vi "canDataSort.vi"() -> ()   [LabVIEW 2023] (continued)
FF\tFF\tFF\tFF\t8C\r\n      1392  1FFFFFFF   00000004    8        00\t00\tFF\tFF\tFF\tFF\tFF\tFF\r\n      1383  0CF102A7   00000004    8        30\t75\tE0\t2E\t80\tFF\tFF\tFD\r\n      1383  0CF101A7   00000004    8        68\t00\t97\tCC\t00\t16\t39\t5F\r\n      1382  1FFFFFFF   00000004    8        00\t00\tFF\tFF\tFF\tFF\tFF\tFF\r\n      1372  1FFFFFFF   00000004    8        00\t00\tFF\tFF\tFF\tFF\tFF\tFF\r\n      1363  0CF102A7   00000004    8        30\t75\tE0\t2E\t80\tFF\tFF\tFD\r\n      1363  0CF101A7   00000004    8        68\t00\t97\tCC\t00\t16\t39\t5E\r\n      1362  1FFFFFFF   00000004    8        00\t00\tFF\tFF\tFF\tFF\tFF\tFF\r\n      1403  0CF102A7   00000004    8        30\t75\tE0\t2E\t80\tFF\tFF\tFD\r\n      1403  0CF101A7   00000004    8        68\t00\t97\tCC\t00\t16\t39\t60\r\n      1402  1FFFFFFF   00000004    8        00\t00\tFF\tFF\tFF\tFF\tFF\tFF\r\n      1393  18F106A7   00000004    8        00\tF7\tFF\tFF\tFF\tFF\tFF\t8C\r\n      1392  1FFFFFFF   00000004    8        00\t00\tFF\tFF\tFF\tFF\tFF\tFF\r\n      1383  0CF102A7   00000004    8        30\t75\tE0\t2E\t80\tFF\tFF\tFD\r\n      1383  0CF101A7   00000004    8        68\t00\t97\tCC\t00\t16\t39\t5F\r\n      1382  1FFFFFFF   00000004    8        00\t00\tFF\tFF\tFF\tFF\tFF\tFF\r\n      1372  1FFFFFFF   00000004    8        00\t00\tFF\tFF\tFF\tFF\tFF\tFF\r\n      1363  0CF102A7   00000004    8        30\t75\tE0\t2E\t80\tFF\tFF\tFD\r\n      1363  0CF101A7   00000004    8        68\t00\t97\tCC\t00\t16\t39\t5E\r\n      1412  1FFFFFFF   00000004    8        00\t00\tFF\tFF\tFF\tFF\tFF\tFF\r\n      1403  0CF102A7   00000004    8        30\t75\tE0\t2E\t80\tFF\tFF\tFD\r\n      1403  0CF101A7   00000004    8        68\t00\t97\tCC\t00\t16\t39\t60\r\n      1402  1FFFFFFF   00000004    8        00\t00\tFF\tFF\tFF\tFF\tFF\tFF\r\n      1393  18F106A7   00000004    8        00\tF7\tFF\tFF\tFF\tFF\tFF\t8C\r\n      1392  1FFFFFFF   00000004    8        00\t00\tFF\tFF\tFF\tFF\tFF\tFF\r\n      1383  0CF102A7   00000004    8        30\t75\tE0\t2E\t80\tFF\tFF\tFD\r\n      1383  0CF101A7   00000004    8        68\t00\t97\tCC\t00\t16\t39\t5F\r\n      1382  1FFFFFFF   00000004    8        00\t00\tFF\tFF\tFF\tFF\tFF\tFF\r\n      1372  1FFFFFFF   00000004    8        00\t00\tFF\tFF\tFF\tFF\tFF\tFF\r\n      1363  0CF102A7   00000004    8        30\t75\tE0\t2E\t80\tFF\tFF\tFD\r\n      1422  1FFFFFFF   00000004    8        00\t00\tFF\tFF\tFF\tFF\tFF\tFF\r\n      1412  1FFFFFFF   00000004    8        00\t00\tFF\tFF\tFF\tFF\tFF\tFF\r\n      1403  0CF102A7   00000004    8        30\t75\tE0\t2E\t80\tFF\tFF\tFD\r\n      1403  0CF101A7   00000004    8        68\t00\t97\tCC\t00\t16\t39\t60\r\n      1402  1FFFFFFF   00000004    8        00\t00\tFF\tFF\tFF\tFF\tFF\tFF\r\n      1393  18F106A7   00000004    8        00\tF7\tFF\tFF\tFF\tFF\tFF\t8C\r\n      1392  1FFFFFFF   00000004    8        00\t00\tFF\tFF\tFF\tFF\tFF\tFF\r\n      1383  0CF102A7   00000004    8        30\t75\tE0\t2E\t80\tFF\tFF\tFD\r\n      1383  0CF101A7   00000004    8        68\t00\t97\tCC\t00\t16\t39\t5F\r\n      1382  1FFFFFFF   00000004    8        00\t00\tFF\tFF\tFF\tFF\tFF\tFF\r\n      1372  1FFFFFFF   00000004    8        00\t00\tFF\tFF\tFF\tFF\tFF\tFF\r\n      1423  0CF101A7   00000004    8        68\t00\t97\tCC\t00\t16\t39\t61\r\n      1422  1FFFFFFF   00000004    8        00\t00\tFF\tFF\tFF\tFF\tFF\tFF\r\n      1412  1FFFFFFF   00000004    8        00\t00\tFF\tFF\tFF\tFF\tFF\tFF\r\n      1403  0CF102A7   00000004    8        30\t75\tE0\t2E\t80\tFF\tFF\tFD\r\n      1403  0CF101A7   00000004    8        68\t00\t97\tCC\t00\t16\t39\t60\r\n      1402  1FFFFFFF   00000004    8        00\t00\tFF\tFF\tFF\tFF\tFF\tFF\r\n      1393  18F106A7   00000004    8        00\tF7\tFF\tFF\tFF\tFF\tFF\t8C\r\n      1392  1FFFFFFF   00000004    8        00\t00\tFF\tFF\tFF\tFF\tFF\tFF\r\n      1383  0CF102A7   00000004    8        30\t75\tE0\t2E\t80\tFF\tFF\tFD\r\n      1383  0CF101A7   00000004    8        68\t00\t97\tCC\t00\t16\t39\t5F\r\n      1382  1FFFFFFF   00000004    8        00\t00\tFF\tFF\tFF\tFF\tFF\tFF\r\n      1423  0CF102A7   00000004    8        30\t75\tE0\t2E\t80\tFF\tFF\tFD\r\n      1423  0CF101A7   00000004    8        68\t00\t97\tCC\t00\t16\t39\t61\r\n      1422  1FFFFFFF   00000004    8        00\t00\tFF\tFF\tFF\tFF\tFF\tFF\r\n      1412  1FFFFFFF   00000004    8        00\t00\tFF\tFF\tFF\tFF\tFF\tFF\r\n      1403  0CF102A7   00000004    8        30\t75\tE0\t2E\t80\tFF\tFF\tFD\r\n      1403  0CF101A7   00000004    8        68\t00\t97\tCC\t00\t16\t39\t60\r\n      1402  1FFFFFFF   00000004    8        00\t00\tFF\tFF\tFF\tFF\tFF\tFF\r\n      1393  18F106A7   00000004    8        00\tF7\tFF\tFF\tFF\tFF\tFF\t8C\r\n      1392  1FFFFFFF   00000004    8        00\t00\tFF\tFF\tFF\tFF\tFF\tFF\r\n      1383  0CF102A7   00000004    8        30\t75\tE0\t2E\t80\tFF\tFF\tFD\r\n      1383  0CF101A7   00000004    8        68\t00\t97\tCC\t00\t16\t39\t5F\r\n      1432  1FFFFFFF   00000004    8        00\t00\tFF\tFF\tFF\tFF\tFF\tFF\r\n      1423  0CF102A7   00000004    8        30\t75\tE0\t2E\t80\tFF\tFF\tFD\r\n      1423  0CF101A7   00000004    8        68\t00\t97\tCC\t00\t16\t39\t61\r\n      1422  1FFFFFFF   00000004    8        00\t00\tFF\tFF\tFF\tFF\tFF\tFF\r\n      1412  1FFFFFFF   00000004    8        00\t00\tFF\tFF\tFF\tFF\tFF\tFF\r\n      1403  0CF102A7   00000004    8        30\t75\tE0\t2E\t80\tFF\tFF\tFD\r\n      1403  0CF101A7   00000004    8        68\t00\t97\tCC\t00\t16\t39\t60\r\n      1402  1FFFFFFF   00000004    8        00\t00\tFF\tFF\tFF\tFF\tFF\tFF\r\n      1393  18F106A7   00000004    8        00\tF7\tFF\tFF\tFF\tFF\tFF\t8C\r\n      1392  1FFFFFFF   00000004    8        00\t00\tFF\tFF\tFF\tFF\tFF\tFF\r\n      1383  0CF102A7   00000004    8        30\t75\tE0\t2E\t80\tFF\tFF\tFD\r\n      1441  18F11FF0   00000004    8        FF\t3F\t90\t68\t88\t1B\t10\t6C\r\n      1432  1FFFFFFF   00000004    8        00\t00\tFF\tFF\tFF\tFF\tFF\tFF\r\n      1423  0CF102A7   00000004    8        30\t75\tE0\t2E\t80\tFF\tFF\tFD\r\n      1423  0CF101A7   00000004    8        68\t00\t97\tCC\t00\t16\t39\t61\r\n      1422  1FFFFFFF   00000004    8        00\t00\tFF\tFF\tFF\tFF\tFF\tFF\r\n      1412  1FFFFFFF   00000004    8        00\t00\tFF\tFF\tFF\tFF\tFF\tFF\r\n      1403  0CF102A7   00000004    8        30\t75\tE0\t2E\t80\tFF\tFF\tFD\r\n      1403  0CF101A7   00000004    8        68\t00\t97\tCC\t00\t16\t39\t60\r\n      1402  1FFFFFFF   00000004    8        00\t00\tFF\tFF\tFF\tFF\tFF\tFF\r\n      1393  18F106A7   00000004    8        00\tF7\tFF\tFF\tFF\tFF\tFF\t8C\r\n      1392  1FFFFFFF   00000004    8        00\t00\tFF\tFF\tFF\tFF\tFF\tFF\r\n      1442  18F120F0   00000004    8        2B\t75\t60\tB1\tB0\t01\tFF\tFF\r\n      1441  18F11FF0   00000004    8        FF\t3F\t90\t68\t88\t1B\t10\t6C\r\n      1432  1FFFFFFF   00000004    8        00\t00\tFF\tFF\tFF\tFF\tFF\tFF\r\n      1423  0CF102A7   00000004    8        30\t75\tE0\t2E\t80\tFF\tFF\tFD\r\n      1423  0CF101A7   00000004    8        68\t00\t97\tCC\t00\t16\t39\t61\r\n      1422  1FFFFFFF   00000004    8        00\t00\tFF\tFF\tFF\tFF\tFF\tFF\r\n      1412  1FFFFFFF   00000004    8        00\t00\tFF\tFF\tFF\tFF\tFF\tFF\r\n      1403  0CF102A7   00000004    8        30\t75\tE0\t2E\t80\tFF\tFF\tFD\r\n      1403  0CF101A7   00000004    8        68\t00\t97\tCC\t00\t16\t39\t60\r\n      1402  1FFFFFFF   00000004    8        00\t00\tFF\tFF\tFF\tFF\tFF\tFF\r\n      1393  18F106A7   00000004    8        00\tF7\tFF\tFF\tFF\tFF\tFF\t8C\r\n      1443  0CF101A7   00000004    8        68\t00\t97\tCC\t00\t16\t39\t62\r\n      1442  18F120F0   00000004    8        2B\t75\t60\tB1\tB0\t01\tFF\tFF\r\n      1441  18F11FF0   00000004    8        FF\t3F\t90\t68\t88\t1B\t10\t6C\r\n      1432  1FFFFFFF   00000004    8        00\t00\tFF\tFF\tFF\tFF\tFF\tFF\r\n      1423  0CF102A7   00000004    8        30\t75\tE0\t2E\t80\tFF\tFF\tFD\r\n      1423  0CF101A7   00000004    8        68\t00\t97\tCC\t00\t16\t39\t61\r\n      1422  1FFFFFFF   00000004    8        00\t00\tFF\tFF\tFF\tFF\tFF\tFF\r\n      1412  1FFFFFFF   00000004    8        00\t00\tFF\tFF\tFF\tFF\tFF\tFF\r\n      1403  0CF102A7   00000004    8        30\t75\tE0\t2E\t80\tFF\tFF\tFD\r\n      1403  0CF101A7   00000004    8        68\t00\t97\tCC\t00\t16\t39\t60\r\n      1402  1FFFFFFF   00000004    8        00\t00\tFF\tFF\tFF\tFF\tFF\tFF\r\n      1443  0C3C4D4A   00000004    8        BE\tFF\tFF\t7F\t18\tFF\tFF\t46\r\n      1443  0CF101A7   00000004    8        68\t00\t97\tCC\t00\t16\t39\t62\r\n      1442  18F120F0   00000004    8        2B\t75\t60\tB1\tB0\t01\tFF\tFF\r\n      1441  18F11FF0   00000004    8        FF\t3F\t90\t68\t88\t1B\t10\t6C\r\n      1432  1FFFFFFF   00000004    8        00\t00\tFF\tFF\tFF\tFF\tFF\tFF\r\n      1423  0CF102A7   00000004    8        30\t75\tE0\t2E\t80\tFF\tFF\tFD\r\n      1423  0CF101A7   00000004    8        68\t00\t97\tCC\t00\t16\t39\t61\r\n      1422  1FFFFFFF   00000004    8        00\t00\tFF\tFF\tFF\tFF\tFF\tFF\r\n      1412  1FFFFFFF   00000004    8        00\t00\tFF\tFF\tFF\tFF\tFF\tFF\r\n      1403  0CF102A7   00000004    8        30\t75\tE0\t2E\t80\tFF\tFF\tFD\r\n      1403  0CF101A7   00000004    8        68\t00\t97\tCC\t00\t16\t39\t60\r\n      1444  0CF102A7   00000004    8        30\t75\tE0\t2E\t80\tFF\tFF\tFD\r\n      1443  0C3C4D4A   00000004    8        BE\tFF\tFF\t7F\t18\tFF\tFF\t46\r\n      1443  0CF101A7   00000004    8        68\t00\t97\tCC\t00\t16\t39\t62\r\n      1442  18F120F0   00000004    8        2B\t75\t60\tB1\tB0\t01\tFF\tFF\r\n      1441  18F11FF0   00000004    8        FF\t3F\t90\t68\t88\t1B\t10\t6C\r\n      1432  1FFFFFFF   00000004    8        00\t00\tFF\tFF\tFF\tFF\tFF\tFF\r\n      1423  0CF102A7   00000004    8        30\t75\tE0\t2E\t80\tFF\tFF\tFD\r\n      1423  0CF101A7   00000004    8        68\t00\t97\tCC\t00\t16\t39\t61\r\n      1422  1FFFFFFF   00000004    8        00\t00\tFF\tFF\tFF\tFF\tFF\tFF\r\n      1412  1FFFFFFF   00000004    8        00\t00\tFF\tFF\tFF\tFF\tFF\tFF\r\n      1403  0CF102A7   00000004    8        30\t75\tE0\t2E\t80\tFF\tFF\tFD\r\n      1444  0CF103A7   00000004    8        17\t1F\t08\t60\tB1\t1F\t08\t46\r\n      1444  0CF102A7   00000004    8        30\t75\tE0\t2E\t80\tFF\tFF\tFD\r\n      1443  0C3C4D4A   00000004    8        BE\tFF\tFF\t7F\t18\tFF\tFF\t46\r\n      1443  0CF101A7   00000004    8        68\t00\t97\tCC\t00\t16\t39\t62\r\n      1442  18F120F0   00000004    8        2B\t75\t60\tB1\tB0\t01\tFF\tFF\r\n      1441  18F11FF0   00000004    8        FF\t3F\t90\t68\t88\t1B\t10\t6C\r\n      1432  1FFFFFFF   00000004    8        00\t00\tFF\tFF\tFF\tFF\tFF\tFF\r\n      1423  0CF102A7   00000004    8        30\t75\tE0\t2E\t80\tFF\tFF\tFD\r\n      1423  0CF101A7   00000004    8        68\t00\t97\tCC\t00\t16\t39\t61\r\n      1422  1FFFFFFF   00000004    8        00\t00\tFF\tFF\tFF\tFF\tFF\tFF\r\n      1412  1FFFFFFF   00000004    8        00\t00\tFF\tFF\tFF\tFF\tFF\tFF\r\n      1445  0CF104A7   00000004    8        F0\t60\t22\tFC\tFF\tFF\tFF\t46\r\n      1444  0CF103A7   00000004    8        17\t1F\t08\t60\tB1\t1F\t08\t46\r\n      1444  0CF102A7   00000004    8        30\t75\tE0\t2E\t80\tFF\tFF\tFD\r\n      1443  0C3C4D4A   00000004    8        BE\tFF\tFF\t7F\t18\tFF\tFF\t46\r\n      1443  0CF101A7   00000004    8        68\t00\t97\tCC\t00\t16\t39\t62\r\n      1442  18F120F0   00000004    8        2B\t75\t60\tB1\tB0\t01\tFF\tFF\r\n      1441  18F11FF0   00000004    8        FF\t3F\t90\t68\t88\t1B\t10\t6C\r\n      1432  1FFFFFFF   00000004    8        00\t00\tFF\tFF\tFF\tFF\tFF\tFF\r\n      1423  0CF102A7   00000004    8        30\t75\tE0\t2E\t80\tFF\tFF\tFD\r\n      1423  0CF101A7   00000004    8        68\t00\t97\tCC\t00\t16\t39\t61\r\n      1422  1FFFFFFF   00000004    8        00\t00\tFF\tFF\tFF\tFF\tFF\tFF\r\n      1445  18F106A7   00000004    8        00\tF7\tFF\tFF\tFF\tFF\tFF\t8D\r\n      1445  0CF104A7   00000004    8        F0\t60\t22\tFC\tFF\tFF\tFF\t46\r\n      1444  0CF103A7   00000004    8        17\t1F\t08\t60\tB1\t1F\t08\t46\r\n      1444  0CF102A7   00000004    8        30\t75\tE0\t2E\t80\tFF\tFF\tFD\r\n      1443  0C3C4D4A   00000004    8        BE\tFF\tFF\t7F\t18\tFF\tFF\t46\r\n      1443  0CF101A7   00000004    8        68\t00\t97\tCC\t00\t16\t39\t62\r\n      1442  18F120F0   00000004    8        2B\t75\t60\tB1\tB0\t01\tFF\tFF\r\n      1441  18F11FF0   00000004    8        FF\t3F\t90\t68\t88\t1B\t10\t6C\r\n      1432  1FFFFFFF   00000004    8        00\t00\tFF\tFF\tFF\tFF\tFF\tFF\r\n      1423  0CF102A7   00000004    8        30\t75\tE0\t2E\t80\tFF\tFF\tFD\r\n      1423  0CF101A7   00000004    8        68\t00\t97\tCC\t00\t16\t39\t61\r\n      1446  18F121F0   00000004    8        09\t18\t00\t00\tFF\tFF\tB0\t01\r\n      1445  18F106A7   00000004    8        00\tF7\tFF\tFF\tFF\tFF\tFF\t8D\r\n      1445  0CF104A7   00000004    8        F0\t60\t22\tFC\tFF\tFF\tFF\t46\r\n      1444  0CF103A7   00000004    8        17\t1F\t08\t60\tB1\t1F\t08\t46\r\n      1444  0CF102A7   00000004    8        30\t75\tE0\t2E\t80\tFF\tFF\tFD\r\n      1443  0C3C4D4A   00000004    8        BE\tFF\tFF\t7F\t18\tFF\tFF\t46\r\n      1443  0CF101A7   00000004    8        68\t00\t97\tCC\t00\t16\t39\t62\r\n      1442  18F120F0   00000004    8        2B\t75\t60\tB1\tB0\t01\tFF\tFF\r\n      1441  18F11FF0   00000004    8        FF\t3F\t90\t68\t88\t1B\t10\t6C\r\n      1432  1FFFFFFF   00000004    8        00\t00\tFF\tFF\tFF\tFF\tFF\tFF\r\n      1423  0CF102A7   00000004    8        30\t75\tE0\t2E\t80\tFF\tFF\tFD\r\n      1447  1FFFFFFF   00000004    8        00\t00\tFF\tFF\tFF\tFF\tFF\tFF\r\n      1446  18F121F0   00000004    8        09\t18\t00\t00\tFF\tFF\tB0\t01\r\n      1445  18F106A7   00000004    8        00\tF7\tFF\tFF\tFF\tFF\tFF\t8D\r\n      1445  0CF104A7   00000004    8        F0\t60\t22\tFC\tFF\tFF\tFF\t46\r\n      1444  0CF103A7   00000004    8        17\t1F\t08\t60\tB1\t1F\t08\t46\r\n      1444  0CF102A7   00000004    8        30\t75\tE0\t2E\t80\tFF\tFF\tFD\r\n      1443  0C3C4D4A   00000004    8        BE\tFF\tFF\t7F\t18\tFF\tFF\t46\r\n      1443  0CF101A7   00000004    8        68\t00\t97\tCC\t00\t16\t39\t62\r\n      1442  18F120F0   00000004    8        2B\t75\t60\tB1\tB0\t01\tFF\tFF\r\n      1441  18F11FF0   00000004    8        FF\t3F\t90\t68\t88\t1B\t10\t6C\r\n      1432  1FFFFFFF   00000004    8        00\t00\tFF\tFF\tFF\tFF\tFF\tFF\r\n      1452  1FFFFFFF   00000004    8        00\t00\tFF\tFF\tFF\tFF\tFF\tFF\r\n      1447  1FFFFFFF   00000004    8        00\t00\tFF\tFF\tFF\tFF\tFF\tFF\r\n      1446  18F121F0   00000004    8        09\t18\t00\t00\tFF\tFF\tB0\t01\r\n      1445  18F106A7   00000004    8        00\tF7\tFF\tFF\tFF\tFF\tFF\t8D\r\n      1445  0CF104A7   00000004    8        F0\t60\t22\tFC\tFF\tFF\tFF\t46\r\n      1444  0CF103A7   00000004    8        17\t1F\t08\t60\tB1\t1F\t08\t46\r\n      1444  0CF102A7   00000004    8        30\t75\tE0\t2E\t80\tFF\tFF\tFD\r\n      1443  0C3C4D4A   00000004    8        BE\tFF\tFF\t7F\t18\tFF\tFF\t46\r\n      1443  0CF101A7   00000004    8        68\t00\t97\tCC\t00\t16\t39\t62\r\n      1442  18F120F0   00000004    8        2B\t75\t60\tB1\tB0\t01\tFF\tFF\r\n      1441  18F11FF0   00000004    8        FF\t3F\t90\t68\t88\t1B\t10\t6C\r\n      1462  1FFFFFFF   00000004    8        00\t00\tFF\tFF\tFF\tFF\tFF\tFF\r\n      1452  1FFFFFFF   00000004    8        00\t00\tFF\tFF\tFF\tFF\tFF\tFF\r\n      1447  1FFFFFFF   00000004    8        00\t00\tFF\tFF\tFF\tFF\tFF\tFF\r\n      1446  18F121F0   00000004    8        09\t18\t00\t00\tFF\tFF\tB0\t01\r\n      1445  18F106A7   00000004    8        00\tF7\tFF\tFF\tFF\tFF\tFF\t8D\r\n      1445  0CF104A7   00000004    8        F0\t60\t22\tFC\tFF\tFF\tFF\t46\r\n      1444  0CF103A7   00000004    8        17\t1F\t08\t60\tB1\t1F\t08\t46\r\n      1444  0CF102A7   00000004    8        30\t75\tE0\t2E\t80\tFF\tFF\tFD\r\n      1443  0C3C4D4A   00000004    8        BE\tFF\tFF\t7F\t18\tFF\tFF\t46\r\n      1443  0CF101A7   00000004    8        68\t00\t97\tCC\t00\t16\t39\t62\r\n      1442  18F120F0   00000004    8        2B\t75\t60\tB1\tB0\t01\tFF\tFF\r\n      1463  0CF101A7   00000004    8        68\t00\t97\tCC\t00\t16\t39\t63\r\n      1462  1FFFFFFF   00000004    8        00\t00\tFF\tFF\tFF\tFF\tFF\tFF\r\n      1452  1FFFFFFF   00000004    8        00\t00\tFF\tFF\tFF\tFF\tFF\tFF\r\n      1447  1FFFFFFF   00000004    8        00\t00\tFF\tFF\tFF\tFF\tFF\tFF\r\n      1446  18F121F0   00000004    8        09\t18\t00\t00\tFF\tFF\tB0\t01\r\n      1445  18F106A7   00000004    8        00\tF7\tFF\tFF\tFF\tFF\tFF\t8D\r\n      1445  0CF104A7   00000004    8        F0\t60\t22\tFC\tFF\tFF\tFF\t46\r\n      1444  0CF103A7   00000004    8        17\t1F\t08\t60\tB1\t1F\t08\t46\r\n      1444  0CF102A7   00000004    8        30\t75\tE0\t2E\t80\tFF\tFF\tFD\r\n      1443  0C3C4D4A   00000004    8        BE\tFF\tFF\t7F\t18\tFF\tFF\t46\r\n      1443  0CF101A7   00000004    8        68\t00\t97\tCC\t00\t16\t39\t62\r\n      1463  0CF102A7   00000004    8        30\t75\tE0\t2E\t80\tFF\tFF\tFD\r\n      1463  0CF101A7   00000004    8        68\t00\t97\tCC\t00\t16\t39\t63\r\n      1462  1FFFFFFF   00000004    8        00\t00\tFF\tFF\tFF\tFF\tFF\tFF\r\n      1452  1FFFFFFF   00000004    8        00\t00\tFF\tFF\tFF\tFF\tFF\tFF\r\n      1447  1FFFFFFF   00000004    8        00\t00\tFF\tFF\tFF\tFF\tFF\tFF\r\n      1446  18F121F0   00000004    8        09\t18\t00\t00\tFF\tFF\tB0\t01\r\n      1445  18F106A7   00000004    8        00\tF7\tFF\tFF\tFF\tFF\tFF\t8D\r\n      1445  0CF104A7   00000004    8        F0\t60\t22\tFC\tFF\tFF\tFF\t46\r\n      1444  0CF103A7   00000004    8        17\t1F\t08\t60\tB1\t1F\t08\t46\r\n      1444  0CF102A7   00000004    8        30\t75\tE0\t2E\t80\tFF\tFF\tFD\r\n      1443  0C3C4D4A   00000004    8        BE\tFF\tFF\t7F\t18\tFF\tFF\t46\r\n      1472  1FFFFFFF   00000004    8        00\t00\tFF\tFF\tFF\tFF\tFF\tFF\r\n      1463  0CF102A7   00000004    8        30\t75\tE0\t2E\t80\tFF\tFF\tFD\r\n      1463  0CF101A7   00000004    8        68\t00\t97\tCC\t00\t16\t39\t63\r\n      1462  1FFFFFFF   00000004    8        00\t00\tFF\tFF\tFF\tFF\tFF\tFF\r\n      1452  1FFFFFFF   00000004    8        00\t00\tFF\tFF\tFF\tFF\tFF\tFF\r\n      1447  1FFFFFFF   00000004    8        00\t00\tFF\tFF\tFF\tFF\tFF\tFF\r\n      1446  18F121F0   00000004    8        09\t18\t00\t00\tFF\tFF\tB0\t01\r\n      1445  18F106A7   00000004    8        00\tF7\tFF\tFF\tFF\tFF\tFF\t8D\r\n      1445  0CF104A7   00000004    8        F0\t60\t22\tFC\tFF\tFF\tFF\t46\r\n      1444  0CF103A7   00000004    8        17\t1F\t08\t60\tB1\t1F\t08\t46\r\n      1444  0CF102A7   00000004    8        30\t75\tE0\t2E\t80\tFF\tFF\tFD\r\n      1482  1FFFFFFF   00000004    8        00\t20\tFF\tFF\tFF\tFF\tFF\tFF\r\n      1472  1FFFFFFF   00000004    8        00\t00\tFF\tFF\tFF\tFF\tFF\tFF\r\n      1463  0CF102A7   00000004    8        30\t75\tE0\t2E\t80\tFF\tFF\tFD\r\n      1463  0CF101A7   00000004    8        68\t00\t97\tCC\t00\t16\t39\t63\r\n      1462  1FFFFFFF   00000004    8        00\t00\tFF\tFF\tFF\tFF\tFF\tFF\r\n      1452  1FFFFFFF   00000004    8        00\t00\tFF\tFF\tFF\tFF\tFF\tFF\r\n      1447  1FFFFFFF   00000004    8        00\t00\tFF\tFF\tFF\tFF\tFF\tFF\r\n      1446  18F121F0   00000004    8        09\t18\t00\t00\tFF\tFF\tB0\t01\r\n      1445  18F106A7   00000004    8        00\tF7\tFF\tFF\tFF\tFF\tFF\t8D\r\n      1445  0CF104A7   00000004    8        F0\t60\t22\tFC\tFF\tFF\tFF\t46\r\n      1444  0CF103A7   00000004    8        17\t1F\t08\t60\tB1\t1F\t08\t46\r\n      1483  0CF101A7   00000004    8        68\t00\t97\tCC\t00\t16\t39\t64\r\n      1482  1FFFFFFF   00000004    8        00\t20\tFF\tFF\tFF\tFF\tFF\tFF\r\n      1472  1FFFFFFF   00000004    8        00\t00\tFF\tFF\tFF\tFF\tFF\tFF\r\n      1463  0CF102A7   00000004    8        30\t75\tE0\t2E\t80\tFF\tFF\tFD\r\n      1463  0CF101A7   00000004    8        68\t00\t97\tCC\t00\t16\t39\t63\r\n      1462  1FFFFFFF   00000004    8        00\t00\tFF\tFF\tFF\tFF\tFF\tFF\r\n      1452  1FFFFFFF   00000004    8        00\t00\tFF\tFF\tFF\tFF\tFF\tFF\r\n      1447  1FFFFFFF   00000004    8        00\t00\tFF\tFF\tFF\tFF\tFF\tFF\r\n      1446  18F121F0   00000004    8        09\t18\t00\t00\tFF\tFF\tB0\t01\r\n      1445  18F106A7   00000004    8        00\tF7\tFF\tFF\tFF\tFF\tFF\t8D\r\n      1445  0CF104A7   00000004    8        F0\t60\t22\tFC\tFF\tFF\tFF\t46\r\n      1483  0CF102A7   00000004    8        30\t75\tE0\t2E\t80\tFF\tFF\tFD\r\n      1483  0CF101A7   00000004    8        68\t00\t97\tCC\t00\t16\t39\t64\r\n      1482  1FFFFFFF   00000004    8        00\t20\tFF\tFF\tFF\tFF\tFF\tFF\r\n      1472  1FFFFFFF   00000004    8        00\t00\tFF\tFF\tFF\tFF\tFF\tFF\r\n      1463  0CF102A7   00000004    8        30\t75\tE0\t2E\t80\tFF\tFF\tFD\r\n      1463  0CF101A7   00000004    8        68\t00\t97\tCC\t00\t16\t39\t63\r\n      1462  1FFFFFFF   00000004    8        00\t00\tFF\tFF\tFF\tFF\tFF\tFF\r\n      1452  1FFFFFFF   00000004    8        00\t00\tFF\tFF\tFF\tFF\tFF\tFF\r\n      1447  1FFFFFFF   00000004    8        00\t00\tFF\tFF\tFF\tFF\tFF\tFF\r\n      1446  18F121F0   00000004    8        09\t18\t00\t00\tFF\tFF\tB0\t01\r\n      1445  18F106A7   00000004    8        00\tF7\tFF\tFF\tFF\tFF\tFF\t8D\r\n      1492  1FFFFFFF   00000004    8        00\t20\tFF\tFF\tFF\tFF\tFF\tFF\r\n      1483  0CF102A7   00000004    8        30\t75\tE0\t2E\t80\tFF\tFF\tFD\r\n      1483  0CF101A7   00000004    8        68\t00\t97\tCC\t00\t16\t39\t64\r\n      1482  1FFFFFFF   00000004    8        00\t20\tFF\tFF\tFF\tFF\tFF\tFF\r\n      1472  1FFFFFFF   00000004    8        00\t00\tFF\tFF\tFF\tFF\tFF\tFF\r\n      1463  0CF102A7   00000004    8        30\t75\tE0\t2E\t80\tFF\tFF\tFD\r\n      1463  0CF101A7   00000004    8        68\t00\t97\tCC\t00\t16\t39\t63\r\n      1462  1FFFFFFF   00000004    8        00\t00\tFF\tFF\tFF\tFF\tFF\tFF\r\n      1452  1FFFFFFF   00000004    8        00\t00\tFF\tFF\tFF\tFF\tFF\tFF\r\n      1447  1FFFFFFF   00000004    8        00\t00\tFF\tFF\tFF\tFF\tFF\tFF\r\n      1446  18F121F0   00000004    8        09\t18\t00\t00\tFF\tFF\tB0\t01\r\n      1493  18F106A7   00000004    8        00\tF7\tFF\tFF\tFF\tFF\tFF\t8E\r\n      1492  1FFFFFFF   00000004    8        00\t20\tFF\tFF\tFF\tFF\tFF\tFF\r\n      1483  0CF102A7   00000004    8        30\t75\tE0\t2E\t80\tFF\tFF\tFD\r\n      1483  0CF101A7   00000004    8        68\t00\t97\tCC\t00\t16\t39\t64\r\n      1482  1FFFFFFF   00000004    8        00\t20\tFF\tFF\tFF\tFF\tFF\tFF\r\n      1472  1FFFFFFF   00000004    8        00\t00\tFF\tFF\tFF\tFF\tFF\tFF\r\n      1463  0CF102A7   00000004    8        30\t75\tE0\t2E\t80\tFF\tFF\tFD\r\n      1463  0CF101A7   00000004    8        68\t00\t97\tCC\t00\t16\t39\t63\r\n      1462  1FFFFFFF   00000004    8        00\t00\tFF\tFF\tFF\tFF\tFF\tFF\r\n      1452  1FFFFFFF   00000004    8        00\t00\tFF\tFF\tFF\tFF\tFF\tFF\r\n      1447  1FFFFFFF   00000004    8        00\t00\tFF\tFF\tFF\tFF\tFF\tFF\r\n      1502  1FFFFFFF   00000004    8        00\t00\tFF\tFF\tFF\tFF\tFF\tFF\r\n      1493  18F106A7   00000004    8        00\tF7\tFF\tFF\tFF\tFF\tFF\t8E\r\n      1492  1FFFFFFF   00000004    8        00\t20\tFF\tFF\tFF\tFF\tFF\tFF\r\n      1483  0CF102A7   00000004    8        30\t75\tE0\t2E\t80\tFF\tFF\tFD\r\n      1483  0CF101A7   00000004    8        68\t00\t97\tCC\t00\t16\t39\t64\r\n      1482  1FFFFFFF   00000004    8        00\t20\tFF\tFF\tFF\tFF\tFF\tFF\r\n      1472  1FFFFFFF   00000004    8        00\t00\tFF\tFF\tFF\tFF\tFF\tFF\r\n      1463  0CF102A7   00000004    8        30\t75\tE0\t2E\t80\tFF\tFF\tFD\r\n      1463  0CF101A7   00000004    8        68\t00\t97\tCC\t00\t16\t39\t63\r\n      1462  1FFFFFFF   00000004    8        00\t00\tFF\tFF\tFF\tFF\tFF\tFF\r\n      1452  1FFFFFFF   00000004    8        00\t00\tFF\tFF\tFF\tFF\tFF\tFF\r\n      1503  0CF101A7   00000004    8        68\t00\t97\tCC\t00\t16\t39\t65\r\n      1502  1FFFFFFF   00000004    8        00\t00\tFF\tFF\tFF\tFF\tFF\tFF\r\n      1493  18F106A7   00000004    8        00\tF7\tFF\tFF\tFF\tFF\tFF\t8E\r\n      1492  1FFFFFFF   00000004    8        00\t20\tFF\tFF\tFF\tFF\tFF\tFF\r\n      1483  0CF102A7   00000004    8        30\t75\tE0\t2E\t80\tFF\tFF\tFD\r\n      1483  0CF101A7   00000004    8        68\t00\t97\tCC\t00\t16\t39\t64\r\n      1482  1FFFFFFF   00000004    8        00\t20\tFF\tFF\tFF\tFF\tFF\tFF\r\n      1472  1FFFFFFF   00000004    8        00\t00\tFF\tFF\tFF\tFF\tFF\tFF\r\n      1463  0CF102A7   00000004    8        30\t75\tE0\t2E\t80\tFF\tFF\tFD\r\n      1463  0CF101A7   00000004    8        68\t00\t97\tCC\t00\t16\t39\t63\r\n      1462  1FFFFFFF   00000004    8        00\t00\tFF\tFF\tFF\tFF\tFF\tFF\r\n      1503  0CF102A7   00000004    8        30\t75\tE0\t2E\t80\tFF\tFF\tFD\r\n      1503  0CF101A7   00000004    8        68\t00\t97\tCC\t00\t16\t39\t65\r\n      1502  1FFFFFFF   00000004    8        00\t00\tFF\tFF\tFF\tFF\tFF\tFF\r\n      1493  18F106A7   00000004    8        00\tF7\tFF\tFF\tFF\tFF\tFF\t8E\r\n      1492  1FFFFFFF   00000004    8        00\t20\tFF\tFF\tFF\tFF\tFF\tFF\r\n      1483  0CF102A7   00000004    8        30\t75\tE0\t2E\t80\tFF\tFF\tFD\r\n      1483  0CF101A7   00000004    8        68\t00\t97\tCC\t00\t16\t39\t64\r\n      1482  1FFFFFFF   00000004    8        00\t20\tFF\tFF\tFF\tFF\tFF\tFF\r\n      1472  1FFFFFFF   00000004    8        00\t00\tFF\tFF\tFF\tFF\tFF\tFF\r\n      1463  0CF102A7   00000004    8        30\t75\tE0\t2E\t80\tFF\tFF\tFD\r\n      1463  0CF101A7   00000004    8        68\t00\t97\tCC\t00\t16\t39\t63\r\n      1512  1FFFFFFF   00000004    8        00\t20\tFF\tFF\tFF\tFF\tFF\tFF\r\n      1503  0CF102A7   00000004    8        30\t75\tE0\t2E\t80\tFF\tFF\tFD\r\n      1503  0CF101A7   00000004    8        68\t00\t97\tCC\t00\t16\t39\t65\r\n      1502  1FFFFFFF   00000004    8        00\t00\tFF\tFF\tFF\tFF\tFF\tFF\r\n      1493  18F106A7   00000004    8        00\tF7\tFF\tFF\tFF\tFF\tFF\t8E\r\n      1492  1FFFFFFF   00000004    8        00\t20\tFF\tFF\tFF\tFF\tFF\tFF\r\n      1483  0CF102A7   00000004    8        30\t75\tE0\t2E\t80\tFF\tFF\tFD\r\n      1483  0CF101A7   00000004    8        68\t00\t97\tCC\t00\t16\t39\t64\r\n      1482  1FFFFFFF   00000004    8        00\t20\tFF\tFF\tFF\tFF\tFF\tFF\r\n      1472  1FFFFFFF   00000004    8        00\t00\tFF\tFF\tFF\tFF\tFF\tFF\r\n      1463  0CF102A7   00000004    8        30\t75\tE0\t2E\t80\tFF\tFF\tFD\r\n      1522  1FFFFFFF   00000004    8        00\t00\tFF\tFF\tFF\tFF\tFF\tFF\r\n      1512  1FFFFFFF   00000004    8        00\t20\tFF\tFF\tFF\tFF\tFF\tFF\r\n      1503  0CF102A7   00000004    8        30\t75\tE0\t2E\t80\tFF\tFF\tFD\r\n      1503  0CF101A7   00000004    8        68\t00\t97\tCC\t00\t16\t39\t65\r\n      1502  1FFFFFFF   00000004    8        00\t00\tFF\tFF\tFF\tFF\tFF\tFF\r\n      1493  18F106A7   00000004    8        00\tF7\tFF\tFF\tFF\tFF\tFF\t8E\r\n      1492  1FFFFFFF   00000004    8        00\t20\tFF\tFF\tFF\tFF\tFF\tFF\r\n      1483  0CF102A7   00000004    8        30\t75\tE0\t2E\t80\tFF\tFF\tFD\r\n      1483  0CF101A7   00000004    8        68\t00\t97\tCC\t00\t16\t39\t64\r\n      1482  1FFFFFFF   00000004    8        00\t20\tFF\tFF\tFF\tFF\tFF\tFF\r\n      1472  1FFFFFFF   00000004    8        00\t00\tFF\tFF\tFF\tFF\tFF\tFF\r\n      1523  0CF101A7   00000004    8        68\t00\t97\tCC\t00\t16\t39\t66\r\n      1522  1FFFFFFF   00000004    8        00\t00\tFF\tFF\tFF\tFF\tFF\tFF\r\n      1512  1FFFFFFF   00000004    8        00\t20\tFF\tFF\tFF\tFF\tFF\tFF\r\n      1503  0CF102A7   00000004    8        30\t75\tE0\t2E\t80\tFF\tFF\tFD\r\n      1503  0CF101A7   00000004    8        68\t00\t97\tCC\t00\t16\t39\t65\r\n      1502  1FFFFFFF   00000004    8        00\t00\tFF\tFF\tFF\tFF\tFF\tFF\r\n      1493  18F106A7   00000004    8        00\tF7\tFF\tFF\tFF\tFF\tFF\t8E\r\n      1492  1FFFFFFF   00000004    8        00\t20\tFF\tFF\tFF\tFF\tFF\tFF\r\n      1483  0CF102A7   00000004    8        30\t75\tE0\t2E\t80\tFF\tFF\tFD\r\n      1483  0CF101A7   00000004    8        68\t00\t97\tCC\t00\t16\t39\t64\r\n      1482  1FFFFFFF   00000004    8        00\t20\tFF\tFF\tFF\tFF\tFF\tFF\r\n      1523  0CF102A7   00000004    8        30\t75\tE0\t2E\t80\tFF\tFF\tFD\r\n      1523  0CF101A7   00000004    8        68\t00\t97\tCC\t00\t16\t39\t66\r\n      1522  1FFFFFFF   00000004    8        00\t00\tFF\tFF\tFF\tFF\tFF\tFF\r\n      1512  1FFFFFFF   00000004    8        00\t20\tFF\tFF\tFF\tFF\tFF\tFF\r\n      1503  0CF102A7   00000004    8        30\t75\tE0\t2E\t80\tFF\tFF\tFD\r\n      1503  0CF101A7   00000004    8        68\t00\t97\tCC\t00\t16\t39\t65\r\n      1502  1FFFFFFF   00000004    8        00\t00\tFF\tFF\tFF\tFF\tFF\tFF\r\n      1493  18F106A7   00000004    8        00\tF7\tFF\tFF\tFF\tFF\tFF\t8E\r\n      1492  1FFFFFFF   00000004    8        00\t20\tFF\tFF\tFF\tFF\tFF\tFF\r\n      1483  0CF102A7   00000004    8        30\t75\tE0\t2E\t80\tFF\tFF\tFD\r\n      1483  0CF101A7   00000004    8        68\t00\t97\tCC\t00\t16\t39\t64\r\n      1532  1FFFFFFF   00000004    8        00\t00\tFF\tFF\tFF\tFF\tFF\tFF\r\n      1523  0CF102A7   00000004    8        30\t75\tE0\t2E\t80\tFF\tFF\tFD\r\n      1523  0CF101A7   00000004    8        68\t00\t97\tCC\t00\t16\t39\t66\r\n      1522  1FFFFFFF   00000004    8        00\t00\tFF\tFF\tFF\tFF\tFF\tFF\r\n      1512  1FFFFFFF   00000004    8        00\t20\tFF\tFF\tFF\tFF\tFF\tFF\r\n      1503  0CF102A7   00000004    8        30\t75\tE0\t2E\t80\tFF\tFF\tFD\r\n      1503  0CF101A7   00000004    8        68\t00\t97\tCC\t00\t16\t39\t65\r\n      1502  1FFFFFFF   00000004    8        00\t00\tFF\tFF\tFF\tFF\tFF\tFF\r\n      1493  18F106A7   00000004    8        00\tF7\tFF\tFF\tFF\tFF\tFF\t8E\r\n      1492  1FFFFFFF   00000004    8        00\t20\tFF\tFF\tFF\tFF\tFF\tFF\r\n      1483  0CF102A7   00000004    8        30\t75\tE0\t2E\t80\tFF\tFF\tFD\r\n      1541  18F11FF0   00000004    8        FF\t3F\t90\t68\t88\t1B\t10\t7C\r\n      1532  1FFFFFFF   00000004    8        00\t00\tFF\tFF\tFF\tFF\tFF\tFF\r\n      1523  0CF102A7   00000004    8        30\t75\tE0\t2E\t80\tFF\tFF\tFD\r\n      1523  0CF101A7   00000004    8        68\t00\t97\tCC\t00\t16\t39\t66\r\n      1522  1FFFFFFF   00000004    8        00\t00\tFF\tFF\tFF\tFF\tFF\tFF\r\n      1512  1FFFFFFF   00000004    8        00\t20\tFF\tFF\tFF\tFF\tFF\tFF\r\n      1503  0CF102A7   00000004    8        30\t75\tE0\t2E\t80\tFF\tFF\tFD\r\n      1503  0CF101A7   00000004    8        68\t00\t97\tCC\t00\t16\t39\t65\r\n      1502  1FFFFFFF   00000004    8        00\t00\tFF\tFF\tFF\tFF\tFF\tFF\r\n      1493  18F106A7   00000004    8        00\tF7\tFF\tFF\tFF\tFF\tFF\t8E\r\n      1492  1FFFFFFF   00000004    8        00\t20\tFF\tFF\tFF\tFF\tFF\tFF\r\n      1542  18F120F0   00000004    8        2B\t75\t60\tB1\tB0\t01\tFF\tFF\r\n      1541  18F11FF0   00000004    8        FF\t3F\t90\t68\t88\t1B\t10\t7C\r\n      1532  1FFFFFFF   00000004    8        00\t00\tFF\tFF\tFF\tFF\tFF\tFF\r\n      1523  0CF102A7   00000004    8        30\t75\tE0\t2E\t80\tFF\tFF\tFD\r\n      1523  0CF101A7   00000004    8        68\t00\t97\tCC\t00\t16\t39\t66\r\n      1522  1FFFFFFF   00000004    8        00\t00\tFF\tFF\tFF\tFF\tFF\tFF\r\n      1512  1FFFFFFF   00000004    8        00\t20\tFF\tFF\tFF\tFF\tFF\tFF\r\n      1503  0CF102A7   00000004    8        30\t75\tE0\t2E\t80\tFF\tFF\tFD\r\n      1503  0CF101A7   00000004    8        68\t00\t97\tCC\t00\t16\t39\t65\r\n      1502  1FFFFFFF   00000004    8        00\t00\tFF\tFF\tFF\tFF\tFF\tFF\r\n      1493  18F106A7   00000004    8        00\tF7\tFF\tFF\tFF\tFF\tFF\t8E\r\n      1543  0CF101A7   00000004    8        68\t00\t97\tCC\t00\t16\t39\t67\r\n      1542  18F120F0   00000004    8        2B\t75\t60\tB1\tB0\t01\tFF\tFF\r\n      1541  18F11FF0   00000004    8        FF\t3F\t90\t68\t88\t1B\t10\t7C\r\n      1532  1FFFFFFF   00000004    8        00\t00\tFF\tFF\tFF\tFF\tFF\tFF\r\n      1523  0CF102A7   00000004    8        30\t75\tE0\t2E\t80\tFF\tFF\tFD\r\n      1523  0CF101A7   00000004    8        68\t00\t97\tCC\t00\t16\t39\t66\r\n      1522  1FFFFFFF   00000004    8        00\t00\tFF\tFF\tFF\tFF\tFF\tFF\r\n      1512  1FFFFFFF   00000004    8        00\t20\tFF\tFF\tFF\tFF\tFF\tFF\r\n      1503  0CF102A7   00000004    8        30\t75\tE0\t2E\t80\tFF\tFF\tFD\r\n      1503  0CF101A7   00000004    8        68\t00\t97\tCC\t00\t16\t39\t65\r\n      1502  1FFFFFFF   00000004    8        00\t00\tFF\tFF\tFF\tFF\tFF\tFF\r\n      1543  0C3C4D4A   00000004    8        BE\tFF\tFF\t7F\t18\tFF\tFF\t47\r\n      1543  0CF101A7   00000004    8        68\t00\t97\tCC\t00\t16\t39\t67\r\n      1542  18F120F0   00000004    8        2B\t75\t60\tB1\tB0\t01\tFF\tFF\r\n      1541  18F11FF0   00000004    8        FF\t3F\t90\t68\t88\t1B\t10\t7C\r\n      1532  1FFFFFFF   00000004    8        00\t00\tFF\tFF\tFF\tFF\tFF\tFF\r\n      1523  0CF102A7   00000004    8        30\t75\tE0\t2E\t80\tFF\tFF\tFD\r\n      1523  0CF101A7   00000004    8        68\t00\t97\tCC\t00\t16\t39\t66\r\n      1522  1FFFFFFF   00000004    8        00\t00\tFF\tFF\tFF\tFF\tFF\tFF\r\n      1512  1FFFFFFF   00000004    8        00\t20\tFF\tFF\tFF\tFF\tFF\tFF\r\n      1503  0CF102A7   00000004    8        30\t75\tE0\t2E\t80\tFF\tFF\tFD\r\n      1503  0CF101A7   00000004    8        68\t00\t97\tCC\t00\t16\t39\t65\r\n      1544  0CF102A7   00000004    8        30\t75\tE0\t2E\t80\tFF\tFF\tFD\r\n      1543  0C3C4D4A   00000004    8        BE\tFF\tFF\t7F\t18\tFF\tFF\t47\r\n      1543  0CF101A7   00000004    8        68\t00\t97\tCC\t00\t16\t39\t67\r\n      1542  18F120F0   00000004    8        2B\t75\t60\tB1\tB0\t01\tFF\tFF\r\n      1541  18F11FF0   00000004    8        FF\t3F\t90\t68\t88\t1B\t10\t7C\r\n      1532  1FFFFFFF   00000004    8        00\t00\tFF\tFF\tFF\tFF\tFF\tFF\r\n      1523  0CF102A7   00000004    8        30\t75\tE0\t2E\t80\tFF\tFF\tFD\r\n      1523  0CF101A7   00000004    8        68\t00\t97\tCC\t00\t16\t39\t66\r\n      1522  1FFFFFFF   00000004    8        00\t00\tFF\tFF\tFF\tFF\tFF\tFF\r\n      1512  1FFFFFFF   00000004    8        00\t20\tFF\tFF\tFF\tFF\tFF\tFF\r\n      1503  0CF102A7   00000004    8        30\t75\tE0\t2E\t80\tFF\tFF\tFD\r\n      1544  0CF103A7   00000004    8        17\t1F\t08\t60\tB1\t1F\t08\t47\r\n      1544  0CF102A7   00000004    8        30\t75\tE0\t2E\t80\tFF\tFF\tFD\r\n      1543  0C3C4D4A   00000004    8        BE\tFF\tFF\t7F\t18\tFF\tFF\t47\r\n      1543  0CF101A7   00000004    8        68\t00\t97\tCC\t00\t16\t39\t67\r\n      1542  18F120F0   00000004    8        2B\t75\t60\tB1\tB0\t01\tFF\tFF\r\n      1541  18F11FF0   00000004    8        FF\t3F\t90\t68\t88\t1B\t10\t7C\r\n      1532  1FFFFFFF   00000004    8        00\t00\tFF\tFF\tFF\tFF\tFF\tFF\r\n      1523  0CF102A7   00000004    8        30\t75\tE0\t2E\t80\tFF\tFF\tFD\r\n      1523  0CF101A7   00000004    8        68\t00\t97\tCC\t00\t16\t39\t66\r\n      1522  1FFFFFFF   00000004    8        00\t00\tFF\tFF\tFF\tFF\tFF\tFF\r\n      1512  1FFFFFFF   00000004    8        00\t20\tFF\tFF\tFF\tFF\tFF\tFF\r\n      1545  0CF104A7   00000004    8        F0\t60\t22\tFC\tFF\tFF\tFF\t47\r\n      1544  0CF103A7   00000004    8        17\t1F\t08\t60\tB1\t1F\t08\t47\r\n      1544  0CF102A7   00000004    8        30\t75\tE0\t2E\t80\tFF\tFF\tFD\r\n      1543  0C3C4D4A   00000004    8        BE\tFF\tFF\t7F\t18\tFF\tFF\t47\r\n      1543  0CF101A7   00000004    8        68\t00\t97\tCC\t00\t16\t39\t67\r\n      1542  18F120F0   00000004    8        2B\t75\t60\tB1\tB0\t01\tFF\tFF\r\n      1541  18F11FF0   00000004    8        FF\t3F\t90\t68\t88\t1B\t10\t7C\r\n      1532  1FFFFFFF   00000004    8        00\t00\tFF\tFF\tFF\tFF\tFF\tFF\r\n      1523  0CF102A7   00000004    8        30\t75\tE0\t2E\t80\tFF\tFF\tFD\r\n      1523  0CF101A7   00000004    8        68\t00\t97\tCC\t00\t16\t39\t66\r\n      1522  1FFFFFFF   00000004    8        00\t00\tFF\tFF\tFF\tFF\tFF\tFF\r\n      1545  18F106A7   00000004    8        00\tF7\tFF\tFF\tFF\tFF\tFF\t8F\r\n      1545  0CF104A7   00000004    8        F0\t60\t22\tFC\tFF\tFF\tFF\t47\r\n      1544  0CF103A7   00000004    8        17\t1F\t08\t60\tB1\t1F\t08\t47\r\n      1544  0CF102A7   00000004    8        30\t75\tE0\t2E\t80\tFF\tFF\tFD\r\n      1543  0C3C4D4A   00000004    8        BE\tFF\tFF\t7F\t18\tFF\tFF\t47\r\n      1543  0CF101A7   00000004    8        68\t00\t97\tCC\t00\t16\t39\t67\r\n      1542  18F120F0   00000004    8        2B\t75\t60\tB1\tB0\t01\tFF\tFF\r\n      1541  18F11FF0   00000004    8        FF\t3F\t90\t68\t88\t1B\t10\t7C\r\n      1532  1FFFFFFF   00000004    8        00\t00\tFF\tFF\tFF\tFF\tFF\tFF\r\n      1523  0CF102A7   00000004    8        30\t75\tE0\t2E\t80\tFF\tFF\tFD\r\n      1523  0CF101A7   00000004    8        68\t00\t97\tCC\t00\t16\t39\t66\r\n      1546  18F121F0   00000004    8        09\t18\t00\t00\tFF\tFF\tB0\t01\r\n      1545  18F106A7   00000004    8        00\tF7\tFF\tFF\tFF\tFF\tFF\t8F\r\n      1545  0CF104A7   00000004    8        F0\t60\t22\tFC\tFF\tFF\tFF\t47\r\n      1544  0CF103A7   00000004    8        17\t1F\t08\t60\tB1\t1F\t08\t47\r\n      1544  0CF102A7   00000004    8        30\t75\tE0\t2E\t80\tFF\tFF\tFD\r\n      1543  0C3C4D4A   00000004    8        BE\tFF\tFF\t7F\t18\tFF\tFF\t47\r\n      1543  0CF101A7   00000004    8        68\t00\t97\tCC\t00\t16\t39\t67\r\n      1542  18F120F0   00000004    8        2B\t75\t60\tB1\tB0\t01\tFF\tFF\r\n      1541  18F11FF0   00000004    8        FF\t3F\t90\t68\t88\t1B\t10\t7C\r\n      1532  1FFFFFFF   00000004    8        00\t00\tFF\tFF\tFF\tFF\tFF\tFF\r\n      1523  0CF102A7   00000004    8        30\t75\tE0\t2E\t80\tFF\tFF\tFD\r\n      1547  1FFFFFFF   00000004    8        00\t00\tFF\tFF\tFF\tFF\tFF\tFF\r\n      1546  18F121F0   00000004    8        09\t18\t00\t00\tFF\tFF\tB0\t01\r\n      1545  18F106A7   00000004    8        00\tF7\tFF\tFF\tFF\tFF\tFF\t8F\r\n      1545  0CF104A7   00000004    8        F0\t60\t22\tFC\tFF\tFF\tFF\t47\r\n      1544  0CF103A7   00000004    8        17\t1F\t08\t60\tB1\t1F\t08\t47\r\n      1544  0CF102A7   00000004    8        30\t75\tE0\t2E\t80\tFF\tFF\tFD\r\n      1543  0C3C4D4A   00000004    8        BE\tFF\tFF\t7F\t18\tFF\tFF\t47\r\n      1543  0CF101A7   00000004    8        68\t00\t97\tCC\t00\t16\t39\t67\r\n      1542  18F120F0   00000004    8        2B\t75\t60\tB1\tB0\t01\tFF\tFF\r\n      1541  18F11FF0   00000004    8        FF\t3F\t90\t68\t88\t1B\t10\t7C\r\n      1532  1FFFFFFF   00000004    8        00\t00\tFF\tFF\tFF\tFF\tFF\tFF\r\n      1552  1FFFFFFF   00000004    8        00\t00\tFF\tFF\tFF\tFF\tFF\tFF\r\n      1547  1FFFFFFF   00000004    8        00\t00\tFF\tFF\tFF\tFF\tFF\tFF\r\n      1546  18F121F0   00000004    8        09\t18\t00\t00\tFF\tFF\tB0\t01\r\n      1545  18F106A7   00000004    8        00\tF7\tFF\tFF\tFF\tFF\tFF\t8F\r\n      1545  0CF104A7   00000004    8        F0\t60\t22\tFC\tFF\tFF\tFF\t47\r\n      1544  0CF103A7   00000004    8        17\t1F\t08\t60\tB1\t1F\t08\t47\r\n      1544  0CF102A7   00000004    8        30\t75\tE0\t2E\t80\tFF\tFF\tFD\r\n      1543  0C3C4D4A   00000004    8        BE\tFF\tFF\t7F\t18\tFF\tFF\t47\r\n      1543  0CF101A7   00000004    8        68\t00\t97\tCC\t00\t16\t39\t67\r\n      1542  18F120F0   00000004    8        2B\t75\t60\tB1\tB0\t01\tFF\tFF\r\n      1541  18F11FF0   00000004    8        FF\t3F\t90\t68\t88\t1B\t10\t7C\r\n      1562  1FFFFFFF   00000004    8        00\t00\tFF\tFF\tFF\tFF\tFF\tFF\r\n      1552  1FFFFFFF   00000004    8        00\t00\tFF\tFF\tFF\tFF\tFF\tFF\r\n      1547  1FFFFFFF   00000004    8        00\t00\tFF\tFF\tFF\tFF\tFF\tFF\r\n      1546  18F121F0   00000004    8        09\t18\t00\t00\tFF\tFF\tB0\t01\r\n      1545  18F106A7   00000004    8        00\tF7\tFF\tFF\tFF\tFF\tFF\t8F\r\n      1545  0CF104A7   00000004    8        F0\t60\t22\tFC\tFF\tFF\tFF\t47\r\n      1544  0CF103A7   00000004    8        17\t1F\t08\t60\tB1\t1F\t08\t47\r\n      1544  0CF102A7   00000004    8        30\t75\tE0\t2E\t80\tFF\tFF\tFD\r\n      1543  0C3C4D4A   00000004    8        BE\tFF\tFF\t7F\t18\tFF\tFF\t47\r\n      1543  0CF101A7   00000004    8      
